vi "PlaceChild.vi"(0 "reference in":refnum<class "Pgui_Obj.lvclass">, 5 "error in (no error)":errorcluster) -> (14 "reference out":refnum<class "Pgui_Obj.lvclass">, 19 "error out":errorcluster)   [LabVIEW 2019, in "Pgui_Obj.lvclass"]
uses:
  Pgui_Obj.lvclass
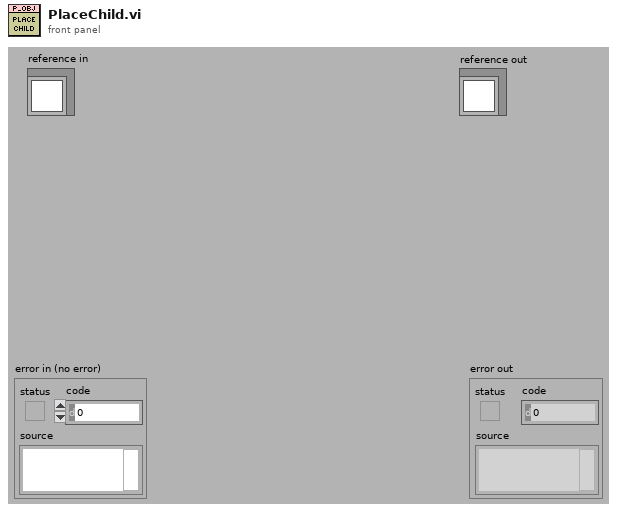
[diagram p1: front panel]
types:
  T1 = typedef "Pgui_Obj.lvclass/ObjectAttributes.ctl" = cluster{"Children":refnum<class "Pgui_Obj.lvclass">[], "Draw Instr":picture, "Params":cluster{"left":i16, "top":i16, "right":i16, "bottom":i16}, "Parent_Pgui_Obj":refnum<class "Pgui_Obj.lvclass">, "MouseOver":bool}
  T2 = cluster{"left":i16, "top":i16, "right":i16, "bottom":i16}
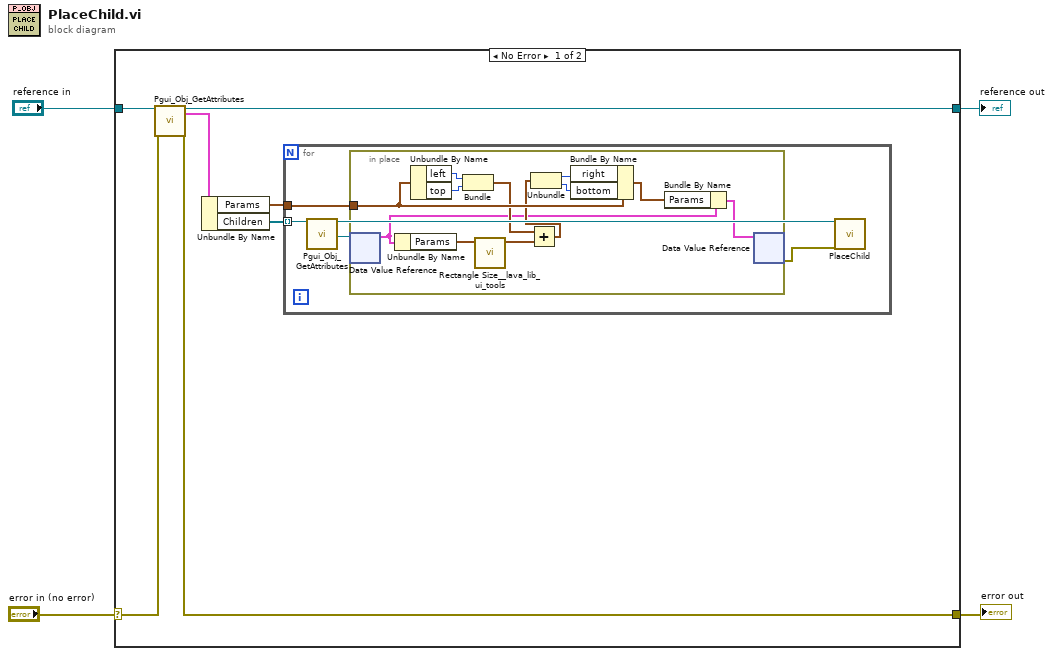
[diagram p0: block diagram]
diagram:
  n1 = case shown="No Error" "error in (no error)" {
    selector: "error in (no error)" -> [w11 w30]
    tunnel: [w9 w30] -> w3
    tunnel: [w7 w29] -> w1
    tunnel: "reference in" -> [w8 w29]
    frame No Error {
      n2 = call "Pgui_Obj_GetAttributes.vi"("reference in"=w8, "error in (no error)"=w11) -> ("reference out"=w7:refnum<class "Pgui_Obj.lvclass">, "Data"=w10:T1, "error out"=w9:errorcluster)  [unwired: 14 in, 1 out]
      n3 = Unbundle By Name(w10) -> ("Params"=w6:T2, "Children"=w5:refnum<class "Pgui_Obj.lvclass">[])
      n4 = for {
        tunnel: w5 -> [w15] mode=indexing
        tunnel: w6 -> [w16]
        n5 = call "Pgui_Obj_GetAttributes.vi"("reference in"=w15) -> ("reference out"=w13:refnum<class "Pgui_Obj.lvclass">, "DataRef"=w14:refnum<data-value>)  [unwired: 15 in, 2 out]
        n6 = in-place {
          in-place-border: w16 -> [w27]
          n7 = in-place-dvr #1(w14) -> (w18:T1)  [unwired: 1 out]
          n8 = Unbundle By Name(w18) -> ("Params"=w28:T2)
          n9 = Unbundle By Name(w27) -> ("left"=w25:i16, "top"=w26:i16)
          n10 = Bundle("left"=w25, "top"=w26) -> (w23:cluster{"left":i16, "top":i16})  [unwired: 1 in]
          n11 = call <vilib>:"Rectangle Size__lava_lib_ui_tools.vi"("Rectangle"=w28) -> ("Rect Size"=w24:cluster{"width":i32, "height":i32})  [unwired: 8 in, 2 out]
          n12 = Add(x=w23, y=w24) -> (x+y=w22:cluster{i32, i32})
          n13 = Unbundle(w22) -> (w21:i32, w20:i32)
          n14 = Bundle By Name(cluster=w27, "right"=w21, "bottom"=w20) -> (w19:T2)
          n15 = Bundle By Name(cluster=w18, "Params"=w19) -> (w17:T1)
          n16 = in-place-dvr #1(w17) -> (w12:errorcluster)  [unwired: 1 out]
        }
        n17 = call-dynamic "PlaceChild.vi"("reference in"=w13, "error in (no error)"=w12) -> ()  [unwired: 16 in, 2 out]
      }
    }
    frame Error {
    }
  }
  "error out" <- w3
  "reference out" <- w1
